vi "run sequence get.vi"(7 "Which Data Technique":T1, 8 "error in":errorcluster) -> (0 "error out":errorcluster, 9 "path":path=path "C:/Documents and Settings/kubley.ONEPURDUE/Desktop/data analysis/modules/sequence calculation")   [LabVIEW 2016]
doc: "on user selection, determines which technique to calculate into sequence results"
uses:
  controls/sequence calculation technique.ctl
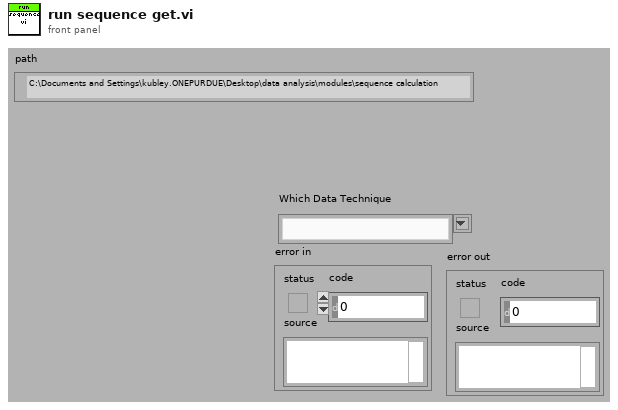
[diagram p1: front panel]
types:
  T1 = typedef "sequence calculation technique.ctl" = string
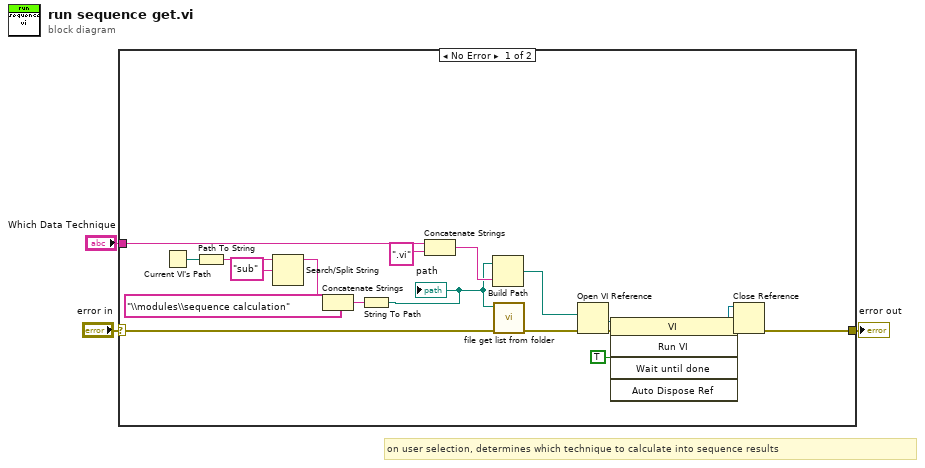
[diagram p0: block diagram]
diagram:
  # "on user selection, determines which technique to calculate into sequence results"
  n1 = case shown="No Error" "error in" {
    selector: "error in" -> [w11 w23]
    tunnel: "Which Data Technique" -> [w15 _]
    tunnel: [w14 w23] -> w2
    frame No Error {
      n2 = Current VI's Path() -> (path=w10:path)
      n3 = Path To String(path=w10) -> (string=w9:string)
      n4 = Search/Split String(string=w9, search string/char (-)="sub") -> (substring before match=w7:string)  [unwired: 1 in, 2 out]
      n5 = Concatenate Strings(w7, "\\modules\\sequence calculation" ("string")) -> (w5:string)
      n6 = String To Path(string=w5) -> (path=w4:path)
      "path" <- w4
      n7 = Concatenate Strings(w15, ".vi" ("string")) -> (w17:string)
      n8 = Build Path(base path=w4, name or relative path=w17) -> (appended path=w12:path)
      n9 = call "file get list from folder.vi"("error in"=w11, "path"=w4) -> ("error out"=w13:errorcluster)  [unwired: 8 in, 1 out]
      n10 = Open VI Reference(vi path=w12, error in (no error)=w13) -> (vi reference=w18:refnum<vi>, error out=w21:errorcluster)  [unwired: 4 in]
      n11 = invoke class="VI" method="Run VI"(reference=w18, error in=w21, "Wait until done"=TRUE ("Wait Until Done")) -> (reference out=w19:refnum<vi>, error out=w20:errorcluster)  [unwired: 2 in, 3 out]
      n12 = Close Reference(reference=w19, error in (no error)=w20) -> (error out=w14:errorcluster)
    }
    frame Error {
    }
  }
  "error out" <- w2
